vi "SIM resample BDs.vi"(8 "Backward differences":dbl[][](array[numeric]), 9 "interp poly order":i32, 10 "current timestep":dbl, 11 "new timestep":dbl) -> (0 "New Backward differences":dbl[][](array[numeric]))   [LabVIEW 2017]
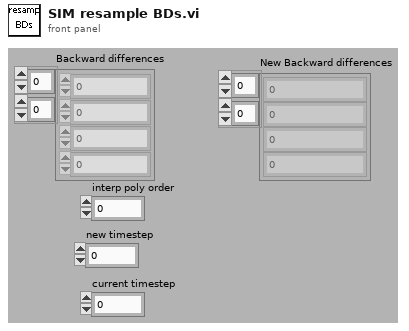
[diagram p1: front panel]
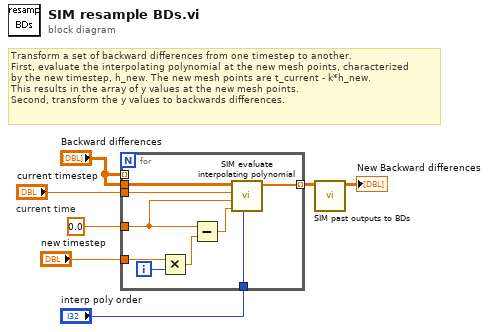
[diagram p0: block diagram]
diagram:
  w5 = 0.0  # current time
  # "Transform a set of backward differences from one timestep to another.\nFirst, evaluate the interpolating polynomial at the new mesh points, characterized\nby the new timestep, h_new. The new mesh points are t_current - k*h_new.\nThis results in the array of y values at the new mesh points. \nSecond, transform the y values to backwards differences."
  n1 = for {
    tunnel: "Backward differences" -> [_] mode=indexing
    tunnel: "Backward differences" -> [w16]
    tunnel: "current timestep" -> [w15]
    tunnel: w5 -> [w14]
    tunnel: "new timestep" -> [w12]
    tunnel: [w9] -> w3 mode=indexing
    tunnel: "interp poly order" -> [w8]
    i -> [w13]
    n2 = Multiply(x=w12, y=w13) -> (x*y=w11:dbl)
    n3 = Subtract(x=w14, y=w11) -> (x-y=w10:dbl)
    n4 = call "SIM evaluate interpolating polynomial.vi"("interp poly order"=w8, "time to evalulate"=w10, "current time"=w14, "timestep"=w15, "Backward differences"=w16) -> ("result"=w9:dbl[])  [unwired: 6 out]
  }
  n5 = call "SIM past outputs to BDs.vi"("Array of previous outputs"=w3) -> ("Corresponding backward differences"=→"New Backward differences":dbl[][])  [unwired: 10 out]
